vi "HEWH GEA2 Loop.vi"() -> ()   [LabVIEW 2016]
uses:
  Washer HCC/Washer HCC NEWFI/Type Definitions/ViperHawk/ViperHawk Data.ctl
  Washer HCC/Washer HCC NEWFI/Type Definitions/ViperHawk/ViperHawk Diagnostic Data.ctl
  Utility/Save File/Public/Type Definitions/Save File Software Version.ctl
  Washer HCC/Washer HCC NEWFI/Type Definitions/ViperHawk/ViperHawk Search Control.ctl
  C:/Technology Lab/NI-2010/Trunk/Utility/LabVIEW GEA2 Toolkit v1.0.0.0/Appliance.NET/GeaCommunication.dll
  Utility/LabVIEW GEA2 Toolkit v1.0.0.0/Appliance.NET/GeaCommunication.dll
  Utility/LabVIEW GEA2 Toolkit v1.0.0.0/type defs/Data Out.ctl
  Utility/GEA2 Commands/HEWH/Type Definitions/GEA2 Commands WaterHeater GEA2 Data.ctl
  Utility/GEA2 Commands/HEWH/Type Definitions/GEA2 Commands Button Status.ctl
  Utility/GEA2 Commands/HEWH/Type Definitions/GEA2 Commands Status Query.ctl
  Utility/GEA2 Commands/HEWH/Type Definitions/GEA2 Commands Service Error Codes.ctl
  Utility/GEA2 Commands/HEWH/Type Definitions/GEA2 Commands.ctl
  Utility/Save File/File Setup (Public)/Type Definition/Save File DOE LabView Program.ctl
  Utility/LabVIEW GEA2 Toolkit v1.0.0.0/library/GEA2_Toolkit.lvlib
  Utility/Save File/File Setup.lvlib
  Utility/Save File/Save File.lvlib
panel:
  in  "Use ERD Routine":bool
  out "HEWH Appliance Data ERD (Newer Routine)":string[][](array[string])
  in  "Disable EMV ERD":bool=TRUE
  in  "#ERDs per message":i32=15
  in  "Retry Count":i32=5
  in  "Board Index ERD":i32
  out "GEA Information Out (Older Routine)":T1={"GEA Diagnostic Data - Washer"={"Speed (RPM)"=0, "Load Size"=0, "Temperature"=0, "Water Pressure"=0.0, "Detergent"=0, "Fabric Softener"=0, "Tub Direction"="", "Detergent Valve"=FALSE, "Fabric Softener Valve"=FALSE, "Recirculating Pump"=FALSE, "Drain Valve"=FALSE, "Hot Valve"=FALSE, "Cold Valve"=FALSE, "Lid Closed Status"="", "Lid Lock Status"="", "Error Count"=0, "IGBT Temperature (Deg C)"=0, "Motor Speed"=0, "Latched OOB"=0, "Raw OOB"=0, "Plaster Status"=0, "Inverter Power (W)"=0, "Target Speed(BRPM)"=0, "Latched Agitate Motor Temp (Deg C)"=0, "Current Motor Temp (Deg C)"=0, "Profiler Status"="", "Current Inverter Action"="", "Error Codes"="", "Lid Locked"=FALSE, "Lid Closed"=FALSE, "9E Diagnostic Data"={"Total Cycle Time (Min)"=0, "Total Cycle Count (Current)"=0, "Total Error Count"=0, "Machine Error History"=0, "Washer UI History"=0, "Inverter Error History"=0, "Cycle Storage Limit"=0, "Error Storage Limit"=0, "Cycle Pages Supported"=0, "Error Pages Supported"=0, "Inverter Reset Count"=0}, "9F Diagnostic Data"={"Cycle Buffer Index"="", "Page Number"="", "Total Cycle Count"=0, "Delay Start Time"=0, "Stain Selected"="", "Selected Cycle"=0, "eWash"="", "Soil Level"="", "Temperature"="", "Overnight Ready"="", "Spin Setting"="", "Control Lock Status"="", "Stain Remover"="", "Steam Assist"="", "My Cycle"="", "PreWash"="", "Debug Log Enabled"="", "Rinse"="", "Signal Level"="", "PreSoak"=""}}, "Software Version"={"Critical Major SW Version"="", "Critical Minor SW Version"="", "Major SW Version"="", "Minor SW Version"="", "Parametric Data Ver. Major"="", "Parametric Data Ver. Minor"="", "Diagnostics Data Ver. Major"="", "Diagnostics Data Ver. Minor"="", "Current Personality Setting"=""}, "Debug Search Parameters"={"Pause"=["MchStdby", "MchPz", "MchIdl", "Machine Standby", "Machine Pause", "Machine Idle"], "Run"=["MchRn", "Machine Run", "Resume Process"], "EOC"=["EOC"], "Error Codes"=["Error1", "try", "rty", "inverr"]}, "Message Count"=0, "Number of Messages"=0, "Partial Message String"="", "Full Message to Save"="", "Board ID"="", "Board Index"=0, "Source Address"=0, "Destination Address"=0, "Data to send"=[], "ReceivedData"=[], "Debug/GEA Data"=[], "Command"=0, "GEA2 Reference Out"=refnum, "GEA2 Event Registration"=refnum, "Bus Data"="", "GEA Data"=[], "Network Variable Location"=0, "Water Heater GEA2 Data"={"GEA2 Label Array"=[], "PID_PARAMETERS"=[], "SUPPORTED_MODES"=[], "Button Status"={"Switch 1"=FALSE, "Switch 2"=FALSE, "Switch 3"=FALSE, "Switch 4"=FALSE, "Switch 5"=FALSE, "Switch 6"=FALSE, "Switch 7"=FALSE, "Switch 8"=FALSE, "Switch 9"=FALSE, "Switch 10"=FALSE, "Switch 11"=FALSE, "Switch 12"=FALSE, "Switch 13"=FALSE, "Switch 14"=FALSE, "Switch 15"=FALSE, "Switch 16"=FALSE}, "Status Query"={"Days Remaining (For Std Electric and Vacation)"=0, "Unit Status"="", "Current Tank Temp in Deg F"=0, "Current Setpoint in Deg F"=0, "Filter Status (% used)"=0, "Fallback Status (Fallback heating mode)"="", "Fallback Temp"=0, "\"Set Mode\" Selection"=""}, "Service Error Codes"={"Reserved"=FALSE, "Reserved 1"=FALSE, "Reserved 2"=FALSE, "Reserved 3"=FALSE, "Reserved 4"=FALSE, "Reserved 5"=FALSE, "Reserved 6"=FALSE, "Reserved 7"=FALSE, "DataFlash Fail Status"=FALSE, "Stuck Key Fail Status"=FALSE, "Dry Tank Fail Status"=FALSE, "Miswire Fail Status"=FALSE, "Reserved 8"=FALSE, "Reserved 9"=FALSE, "Reserved 10"=FALSE, "Reserved 11"=FALSE, "UE Fail Status"=FALSE, "LE Fail Status"=FALSE, "Filter Fail Status"=FALSE, "T3A Fail Status"=FALSE, "T3B Fail Status"=FALSE, "T4 Fail Status"=FALSE, "T5 Fail Status"=FALSE, "T2 Fail Status"=FALSE, "SS Cond A Status"=FALSE, "SS Cond B Status"=FALSE, "SS Cond C Status"=FALSE, "SS Cond D Status"=FALSE, "SS Cond E Status"=FALSE, "SS Cond F Status"=FALSE, "SS Fan Status"=FALSE, "CMP Fail Status"=FALSE}, "HEM_KWH_DATA"=[], "OTHER_FAULT_COUNTS"=[], "GEA2 Raw Message"="", "Hyperterminal Data"={"Source"=0, "Destination"=0, "Command"=0, "Length"=0, "CRC"=0, "UE - state (1/0 on off)"=0, "LE - state (1/0 on off)"=0, "Comp - state (1/0 on off)"=0, "Fan  - state (1/0 on off)"=0, "Setpoint Deg F"=0, "T2(TankSensor)"=0.0, "T3A(EvapIn)"=0.0, "T3B(EvapOut)"=0.0, "T4(CompressorDischarge)"=0.0, "T5(Ambient)"=0.0, "Current"=0.0, "Voltage (Volts)"=0, "EEV Position (0-480)"=0, "Reason for last heating cycle termination"=0, "Reason Data word 1"="", "Reason Data word 2"="", "Reason Data word 3"="", "Reason Data word 4"="", "SW Debug Data"="", "Flow Events (Bit Encoded)"=0, "Heating Control Mode"=0}, "Extra Data"={"Water Capacity (Gallons)"=0, "Max Vacation Duration Days"=0, "Min Vacation Duration Days"=0, "Max Set Point (Deg F)"=0, "Min Set Point (Deg F)"=0, "T5 Resistance"=0, "T4 Resistance"=0, "T3B Resistance"=0, "T2 Resistance"=0, "STD_ELEC_RANGE"="", "SS_FAULT_COUNTS"="", "SERIAL_NUMBER"="", "READ_PERSONALITY"=0, "RQST_OVERRIDE_STATUS"="", "MODEL_SELECT_AD_VALUE"=0, "MODEL NUMBER"="", "IDLB_RESISTANCE"=0, "DSM Override Status"="", "RQST_DATA_FROM_Memory"="", "RQST_DATA_FROM_DATA_FLASH"="", "RQST_CURRENT_PID_SH_TARGET"=0, "Unit System Mode"=""}}} {"Water Heater GEA2 Data"."Hyperterminal Data"."CRC" format="%x"; "Water Heater GEA2 Data"."Hyperterminal Data"."Length" format="%x"; "Water Heater GEA2 Data"."Hyperterminal Data"."Command" format="%x"; "Water Heater GEA2 Data"."Hyperterminal Data"."Destination" format="%x"; "Water Heater GEA2 Data"."Hyperterminal Data"."Source" format="%x"; "Destination Address" format="%x"; "Source Address" format="%x"; "Command" format="%.0x"; "Data to send" format="%x"; "ReceivedData" format="%x"}
  out "Board ID":string
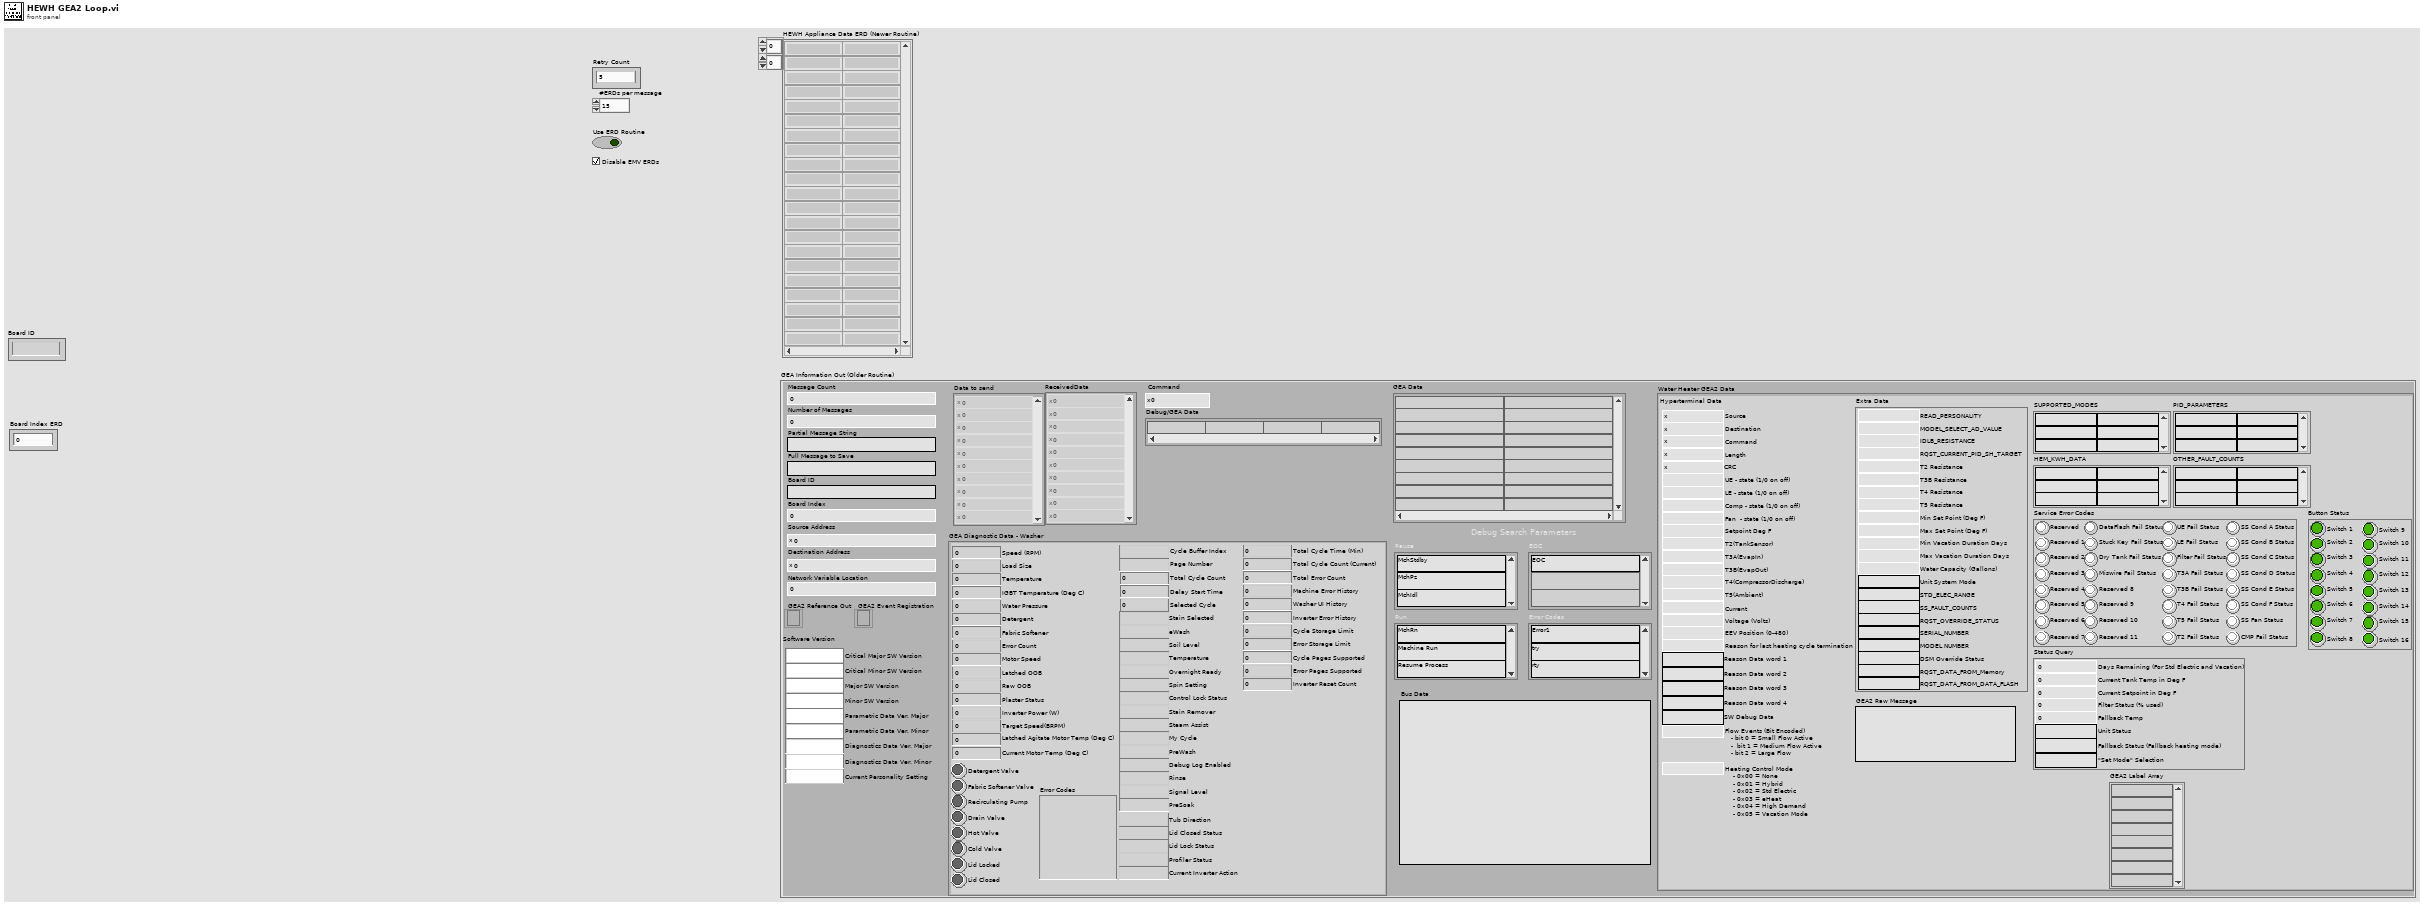
[diagram p1: front panel]
types:
  T1 = typedef "ViperHawk Data.ctl" = cluster{"GEA Diagnostic Data - Washer":T2, "Software Version":T3, "Debug Search Parameters":T4, "Message Count":i32, "Number of Messages":i32, "Partial Message String":string, "Full Message to Save":string, "Board ID":string, "Board Index":i32, "Source Address":u8, "Destination Address":u8, "Data to send":u8[], "ReceivedData":u8[], "Debug/GEA Data":string[], "Command":u8, "GEA2 Reference Out":refnum<k24>, "GEA2 Event Registration":refnum<event-registration>, "Bus Data":string, "GEA Data":string[][], "Network Variable Location":i32, "Water Heater GEA2 Data":T5}
  T2 = typedef "ViperHawk Diagnostic Data.ctl" = cluster{"Speed (RPM)":u32, "Load Size":u32, "Temperature":u32, "Water Pressure":dbl, "Detergent":u32, "Fabric Softener":u32, "Tub Direction":string, "Detergent Valve":bool, "Fabric Softener Valve":bool, "Recirculating Pump":bool, "Drain Valve":bool, "Hot Valve":bool, "Cold Valve":bool, "Lid Closed Status":string, "Lid Lock Status":string, "Error Count":u32, "IGBT Temperature (Deg C)":u32, "Motor Speed":u32, "Latched OOB":u32, "Raw OOB":u32, "Plaster Status":u32, "Inverter Power (W)":u32, "Target Speed(BRPM)":u32, "Latched Agitate Motor Temp (Deg C)":u32, "Current Motor Temp (Deg C)":u32, "Profiler Status":string, "Current Inverter Action":string, "Error Codes":string, "Lid Locked":bool, "Lid Closed":bool, "9E Diagnostic Data":cluster{"Total Cycle Time (Min)":u32, "Total Cycle Count (Current)":u16, "Total Error Count":u16, "Machine Error History":u32, "Washer UI History":u32, "Inverter Error History":u32, "Cycle Storage Limit":u8, "Error Storage Limit":u8, "Cycle Pages Supported":u8, "Error Pages Supported":u8, "Inverter Reset Count":u16}, "9F Diagnostic Data":cluster{"Cycle Buffer Index":string, "Page Number":string, "Total Cycle Count":u32, "Delay Start Time":u32, "Stain Selected":string, "Selected Cycle":u32, "eWash":string, "Soil Level":string, "Temperature":string, "Overnight Ready":string, "Spin Setting":string, "Control Lock Status":string, "Stain Remover":string, "Steam Assist":string, "My Cycle":string, "PreWash":string, "Debug Log Enabled":string, "Rinse":string, "Signal Level":string, "PreSoak":string}}
  T3 = typedef "Save File.lvlib/Save File Software Version.ctl" = cluster{"Critical Major SW Version":string, "Critical Minor SW Version":string, "Major SW Version":string, "Minor SW Version":string, "Parametric Data Ver. Major":string, "Parametric Data Ver. Minor":string, "Diagnostics Data Ver. Major":string, "Diagnostics Data Ver. Minor":string, "Current Personality Setting":string}
  T4 = typedef "ViperHawk Search Control.ctl" = cluster{"Pause":string[], "Run":string[], "EOC":string[], "Error Codes":string[]}
  T5 = typedef "GEA2 Commands WaterHeater GEA2 Data.ctl" = cluster{"GEA2 Label Array":string[], "PID_PARAMETERS":string[][], "SUPPORTED_MODES":string[][], "Button Status":T6, "Status Query":T7, "Service Error Codes":T8, "HEM_KWH_DATA":string[][], "OTHER_FAULT_COUNTS":string[][], "GEA2 Raw Message":string, "Hyperterminal Data":cluster{"Source":u8, "Destination":u8, "Command":u8, "Length":u8, "CRC":u16, "UE - state (1/0 on off)":u8, "LE - state (1/0 on off)":u8, "Comp - state (1/0 on off)":u8, "Fan  - state (1/0 on off)":u8, "Setpoint Deg F":i32, "T2(TankSensor)":dbl, "T3A(EvapIn)":dbl, "T3B(EvapOut)":dbl, "T4(CompressorDischarge)":dbl, "T5(Ambient)":dbl, "Current":dbl, "Voltage (Volts)":u16, "EEV Position (0-480)":u16, "Reason for last heating cycle termination":u16, "Reason Data word 1":string, "Reason Data word 2":string, "Reason Data word 3":string, "Reason Data word 4":string, "SW Debug Data":string, "Flow Events (Bit Encoded)":u16, "Heating Control Mode":u16}, "Extra Data":cluster{"Water Capacity (Gallons)":u32, "Max Vacation Duration Days":u32, "Min Vacation Duration Days":u32, "Max Set Point (Deg F)":u32, "Min Set Point (Deg F)":u32, "T5 Resistance":u32, "T4 Resistance":u32, "T3B Resistance":u32, "T2 Resistance":u32, "STD_ELEC_RANGE":string, "SS_FAULT_COUNTS":string, "SERIAL_NUMBER":string, "READ_PERSONALITY":u8, "RQST_OVERRIDE_STATUS":string, "MODEL_SELECT_AD_VALUE":u32, "MODEL NUMBER":string, "IDLB_RESISTANCE":u32, "DSM Override Status":string, "RQST_DATA_FROM_Memory":string, "RQST_DATA_FROM_DATA_FLASH":string, "RQST_CURRENT_PID_SH_TARGET":u16, "Unit System Mode":string}}
  T6 = typedef "GEA2 Commands Button Status.ctl" = cluster{"Switch 1":bool, "Switch 2":bool, "Switch 3":bool, "Switch 4":bool, "Switch 5":bool, "Switch 6":bool, "Switch 7":bool, "Switch 8":bool, "Switch 9":bool, "Switch 10":bool, "Switch 11":bool, "Switch 12":bool, "Switch 13":bool, "Switch 14":bool, "Switch 15":bool, "Switch 16":bool}
  T7 = typedef "GEA2 Commands Status Query.ctl" = cluster{"Days Remaining (For Std Electric and Vacation)":u8, "Unit Status":string, "Current Tank Temp in Deg F":u8, "Current Setpoint in Deg F":u8, "Filter Status (% used)":u8, "Fallback Status (Fallback heating mode)":string, "Fallback Temp":u8, "\"Set Mode\" Selection":string}
  T8 = typedef "GEA2 Commands Service Error Codes.ctl" = cluster{"Reserved":bool, "Reserved 1":bool, "Reserved 2":bool, "Reserved 3":bool, "Reserved 4":bool, "Reserved 5":bool, "Reserved 6":bool, "Reserved 7":bool, "DataFlash Fail Status":bool, "Stuck Key Fail Status":bool, "Dry Tank Fail Status":bool, "Miswire Fail Status":bool, "Reserved 8":bool, "Reserved 9":bool, "Reserved 10":bool, "Reserved 11":bool, "UE Fail Status":bool, "LE Fail Status":bool, "Filter Fail Status":bool, "T3A Fail Status":bool, "T3B Fail Status":bool, "T4 Fail Status":bool, "T5 Fail Status":bool, "T2 Fail Status":bool, "SS Cond A Status":bool, "SS Cond B Status":bool, "SS Cond C Status":bool, "SS Cond D Status":bool, "SS Cond E Status":bool, "SS Cond F Status":bool, "SS Fan Status":bool, "CMP Fail Status":bool}
  T9 = typedef "GEA2 Commands.ctl" = enum16{"CMD_CANCEL_EEV_POSITION", "CMD_CLEAR_ENERGY_USAGE_CTRS", "CMD_CLEAR_FAULT_COUNTS", "CMD_CLEAR_OVERRIDE_STATUS", "CMD_COMP_OFF", "CMD_COMP_ON", "CMD_DSM_OVERRIDES", "CMD_EEV_POSITION", "CMD_ENTER_EXIT_FCT_MODE", "CMD_ENTER_FACT_MODE", "CMD_HP_RUN_6MIN", "CMD_INITIATE_REMOTE_DSM_OVERRIDE", "CMD_LE_2_SECONDS", "CMD_REFRESH_SERVICE_TIMEOUTS", "CMD_RESET", "CMD_RESET_FILTER_TIMES", "CMD_RESTORE_EEPROM_DEFAULTS", "CMD_RQST_LED_STATUS", "CMD_SET_AMBIENT_THRESH_1", "CMD_SET_AMBIENT_THRESH_2", "CMD_SET_AMBIENT_THRESH_3", "CMD_SET_CURRENTS", "CMD_SET_EEV_DRIVE_LINES", "CMD_SET_EEV_STOP_POSITION", "CMD_SET_LEDS", "CMD_SET_MODEL_NUMBER", "CMD_SET_PID_I_DENOM_OVER_THR", "CMD_SET_PID_I_DENOM_UNDER_THR", "CMD_SET_PID_LOW_SH_TARGET", "CMD_SET_PID_MID_SH_TARGET", "CMD_SET_PID_P_DENOMINATOR", "CMD_SET_SERIAL_NUMBER", "CMD_SET_START_POS_OVER_THR", "CMD_SET_START_POS_UNDER_THR", "CMD_TOGGLE_FAN", "CMD_TOGGLE_LE_SERV", "CMD_TOGGLE_SERVICE_MODE", "CMD_TOGGLE_UE_SERV", "CMD_TURN_ON_OFF_DLB", "CMD_UE_2_SECONDS", "CMD_UPDATE_DSM_LEVEL", "CMD_UPDATE_MODE", "CMD_WRITE_SETPOINTS", "REQ_READ_KEY_STATUS", "REQ_SYSTEM_MODE", "RQST_CURRENT_PID_SH_TARGET", "RQST_DATA_FROM_DATA_FLASH", "RQST_DATA_FROM_MEMORY", "RQST_DSM_OVERRIDE_STATUS", "RQST_HEM_KWH_DATA", "RQST_HYPERTERM_OUTPUT_DATA", "RQST_IDLB_RESISTANCE", "RQST_MODEL_NUMBER", "RQST_MODEL_SELECT_AD_VALUE", "RQST_OTHER_FAULT_COUNTS", "RQST_OVERRIDE_STATUS", "RQST_PID_PARAMETERS", "RQST_READ_PERSONALITY", "RQST_SERIAL_NUMBER", "RQST_SERVICE_ERROR_CODES", "RQST_Software_Version", "RQST_SS_FAULT_COUNTS", "RQST_STATUS_QUERY", "RQST_STD_ELEC_RANGE", "RQST_SUPPORTED_MODES", "RQST_T2_RESISTANCE", "RQST_T3B_RESISTANCE", "RQST_T4_RESISTANCE", "RQST_T5_RESISTANCE", "RQST_TEMP_RANGE", "RQST_VACATION_RANGE", "RQST_WATER_CAPACITY"}
  T10 = typedef "GEA2_Toolkit.lvlib/Data In.ctl" = cluster{"Source":u8, "Destination":u8, "Command":u8, "Message":string}
  T11 = typedef "File Setup.lvlib/Save File DOE LabView Program.ctl" = enum16{"No Name Found", "DOE Stand", "Dishwasher Kitchen", "Portable Stand", "HEWH", "Dryer", "Dryer WILT", "HCC", "PRAT", "HEWH RLT"}
  T12 = typedef "GEA2_Toolkit.lvlib/Data Out.ctl" = cluster{"Source":u8, "Destination":u8, "Command":u8, "Length":u8, "CRC":u16, "Message":string}
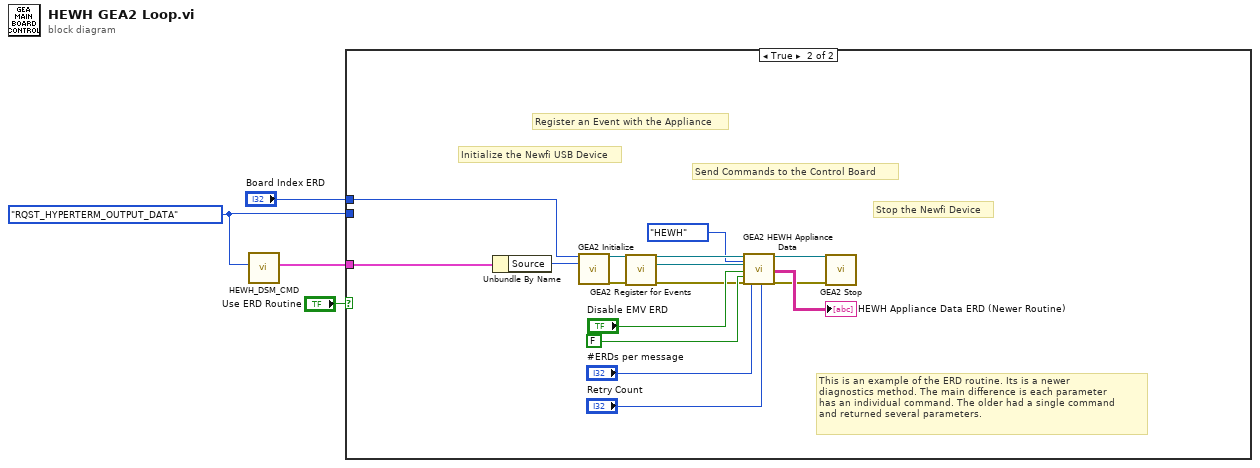
[diagram p0: block diagram]
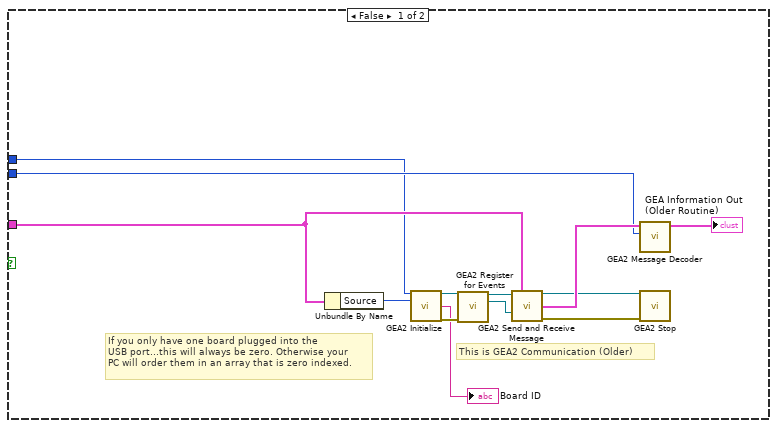
[diagram p2: hidden frame]
diagram:
  w4 = GEA2_Commands."RQST_HYPERTERM_OUTPUT_DATA" ("GEA2 Commands and Requests")
  n1 = call "HEWH_DSM_CMD.vi"("GEA2 Commands and Requests"=w4) -> ("Input Data"=w3:T10)  [unwired: 8 in, 1 out]
  n2 = case shown="True" "Use ERD Routine" {
    tunnel: w4 -> [w7 _]
    tunnel: w3 -> [w6 w19]
    tunnel: "Board Index ERD" -> [w5 w18]
    frame False {
      # "This is GEA2 Communication (Older)"
      # "If you only have one board plugged into the\nUSB port...this will always be zero. Otherwise your \nPC will order them in an array that is zero indexed."
      n3 = Unbundle By Name(w6) -> ("Source"=w10:u8)
      n4 = call "GEA2 Initialize.vi"("Board Index"=w5, "Source Address"=w10) -> ("GEA2 Reference Out"=w14:refnum<k24>, "Board ID"=→"Board ID":string, "error out"=w15:errorcluster)  [unwired: 11 in]
      n5 = call "GEA2 Register for Events.vi"("GEA2 Reference In"=w14, "Error In"=w15) -> ("GEA2 Reference Out"=w16:refnum<k24>, "GEA2 Event Registration"=w17:refnum<event-registration>)  [unwired: 11 in, 1 out]
      n6 = call "GEA2 Send and Receive Message.vi"("GEA2 Reference In"=w16, "Input Data"=w6, "GEA2 Event Registration"=w17) -> ("GEA2 Reference Out"=w8:refnum<k24>, "Converted Data Out"=w11:T12, "Error Out"=w9:errorcluster)  [unwired: 7 in, 3 out]
      n7 = call "GEA2 Message Decoder.vi"("GEA2 Commands and Requests"=w7, "Coverted Data Out"=w11) -> ("GEA Information Out"=→"GEA Information Out (Older Routine)":T1)  [unwired: 9 in]
      n8 = call "GEA2 Stop.vi"("GEA2 Reference Out"=w8, "Error In"=w9) -> ()  [unwired: 13 in, 1 out]
    }
    frame True {
      # "Stop the Newfi Device"
      # "Send Commands to the Control Board"
      # "Register an Event with the Appliance"
      # "Initialize the Newfi USB Device"
      # "This is an example of the ERD routine. Its is a newer \ndiagnostics method. The main difference is each parameter\nhas an individual command. The older had a single command\nand returned several parameters."
      n9 = Unbundle By Name(w19) -> ("Source"=w31:u8)
      n10 = call "GEA2 Initialize.vi"("Board Index"=w18, "Source Address"=w31) -> ("GEA2 Reference Out"=w32:refnum<k24>, "error out"=w33:errorcluster)  [unwired: 11 in, 1 out]
      n11 = call "GEA2 Register for Events.vi"("GEA2 Reference In"=w32, "Error In"=w33) -> ("GEA2 Reference Out"=w30:refnum<k24>, "GEA2 Event Registration"=w29:refnum<event-registration>, "Error Out"=w23:errorcluster)  [unwired: 11 in]
      n12 = call "GEA2 HEWH Appliance Data.vi"(".NET Refnum in"=w30, "LV Program"=Save_File_DOE_LabView_Program."HEWH", "GEA2 Event Registration In"=w29, "Disable Electronic Mixing Valve (EMV) List"="Disable EMV ERD", "Disable Classic GEA2"=FALSE, "error in (no error)"=w23, "#ERDs per message"="#ERDs per message", "Retry Count"="Retry Count") -> (".NET Refnum out"=w20:refnum<k24>, "HEWH Appliance Data ERD"=→"HEWH Appliance Data ERD (Newer Routine)":string[][], "error out"=w21:errorcluster)  [unwired: 5 in, 4 out]
      n13 = call "GEA2 Stop.vi"("GEA2 Reference Out"=w20, "Error In"=w21) -> ()  [unwired: 13 in, 1 out]
    }
  }
